vi "Update List of Controls Tree.vi"(8 "error in (no error)":errorcluster, 11 "Data Cluster":T1) -> (0 "error out":errorcluster, 3 "Items":T2(array[cluster]))   [LabVIEW 2020, in "Control Property Tree.lvlib"]
uses:
  Control Property Tree.lvlib
  Module Data--cluster.ctl
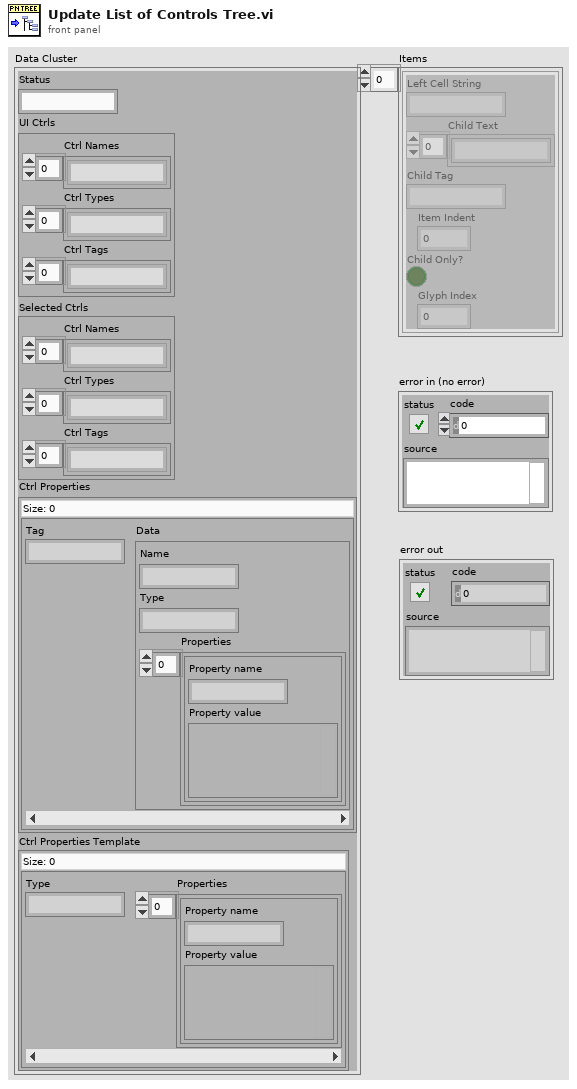
[diagram p1: front panel]
types:
  T1 = typedef "Control Property Tree.lvlib/Module Data--cluster.ctl" = cluster{"Status":string, "UI Ctrls":cluster{"Ctrl Names":string[], "Ctrl Types":string[], "Ctrl Tags":string[]}, "Selected Ctrls":cluster{"Ctrl Names":string[], "Ctrl Types":string[], "Ctrl Tags":string[]}, "Ctrl Properties":map{string, cluster{"Name":string, "Type":string, "Properties":cluster{"Property name":string, "Property value":variant}[]}}, "Ctrl Properties Template":map{string, cluster{"Property name":string, "Property value":variant}[]}}
  T2 = cluster{"Left Cell String":string, "Child Text":string[], "Child Tag":string, "Item Indent":i32, "Child Only?":bool, "Glyph Index":i32}[]
  T3 = cluster{"Left Cell String":string, "Child Text":string[], "Child Tag":string, "Item Indent":i32, "Child Only?":bool, "Glyph Index":i32}
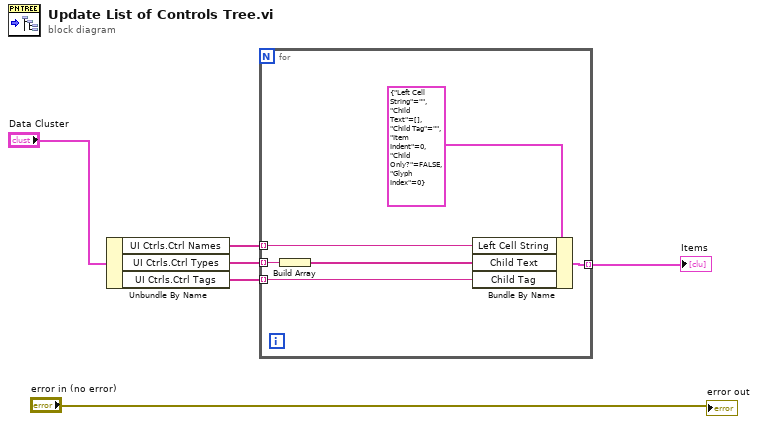
[diagram p0: block diagram]
diagram:
  n1 = Unbundle By Name("Data Cluster") -> ("UI Ctrls.Ctrl Names"=w3:string[], "UI Ctrls.Ctrl Types"=w4:string[], "UI Ctrls.Ctrl Tags"=w5:string[])
  n2 = for {
    tunnel: w3 -> [w10] mode=indexing
    tunnel: w4 -> [w9] mode=indexing
    tunnel: w5 -> [w7] mode=indexing
    tunnel: [w12] -> w6 mode=indexing
    n3 = Build Array(w9) -> (w8:string[])
    n4 = Bundle By Name(cluster=T3 {"Left Cell String"="", "Child Text"=[], "Child Tag"="", "Item Indent"=0, "Child Only?"=FALSE, "Glyph Index"=0} ("Item"), "Left Cell String"=w10, "Child Text"=w8, "Child Tag"=w7) -> (w12:T3)
  }
  "Items" <- w6
  "error out" <- "error in (no error)"
